vi "OEE_SCREEN_2_generate_accumulative_graph_values.vi"(11 "SCREEN_2_graph_accumulative_all_info":T1={"hour_start"=8, "hour_end"=8, "actual_by_hour"=[], "target_by_hour"=[], "X_axis_labels"=[], "SCREEN_2_graph_accumulative_references"={"graph_accumulative"=refnum, "labels_picture_accumulative"=refnum, "front_panel_reference"=refnum}}) -> (1 "Y_scale_max":dbl=160.0, 2 "Y_annotation_offset":dbl=7.9750000000000005, 3 "graph_values":cluster{dbl[], dbl[]}[](array[cluster])=[{[8.5, 9.5, 10.5, 11.5, 12.5, 13.5, 14.5, 15.5, 16.5, 17.5, 18.5, 19.5], [1.0, 5.0, 7.0, 0.0, 0.0, 0.0, 0.0, 0.0, 0.0, 0.0, 0.0, 0.0]}, {[8.5, 9.5, 10.5, 11.5, 12.5, 13.5, 14.5, 15.5, 16.5, 17.5, 18.5, 19.5], [10.0, 20.0, 30.0, 40.0, 50.0, 60.0, 70.0, 80.0, 90.0, 110.0, 120.0, 130.0]}])   [LabVIEW 2019]
uses:
  FGV/FGV_SCREEN_2_graph_accumulative/FGV_SCREEN_2_graph_accumulative_all_info.ctl
  FGV/FGV_SCREEN_2_graph_accumulative/FGV_SCREEN_2_graph_accumulative_references.ctl
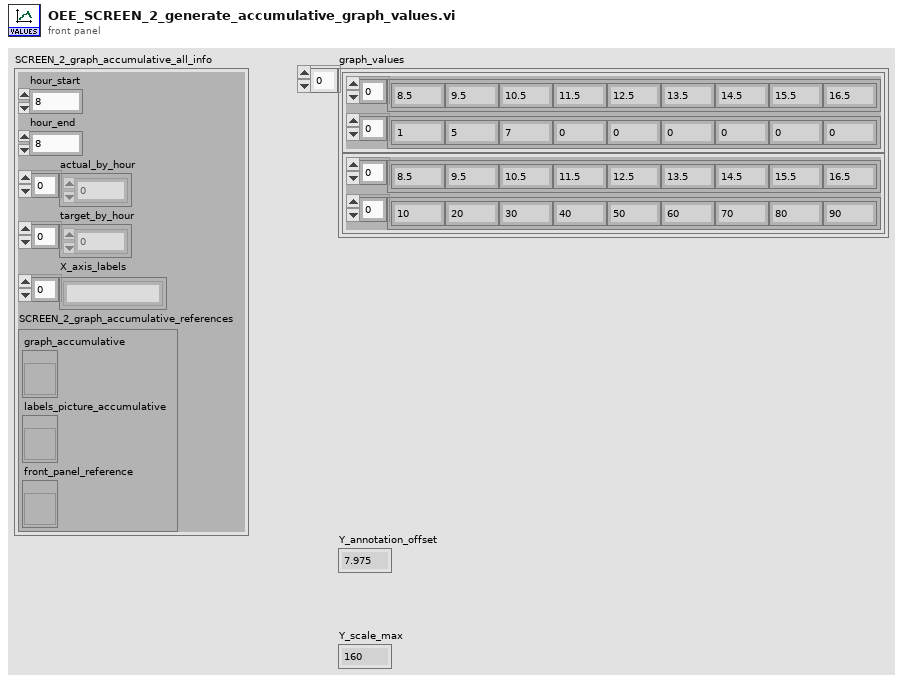
[diagram p1: front panel]
types:
  T1 = typedef "FGV_SCREEN_2_graph_accumulative_all_info.ctl" = cluster{"hour_start":i8, "hour_end":i8, "actual_by_hour":u16[], "target_by_hour":u16[], "X_axis_labels":string[], "SCREEN_2_graph_accumulative_references":T2}
  T2 = typedef "FGV_SCREEN_2_graph_accumulative_references.ctl" = cluster{"graph_accumulative":refnum<vi>, "labels_picture_accumulative":refnum<vi>, "front_panel_reference":refnum<vi>}
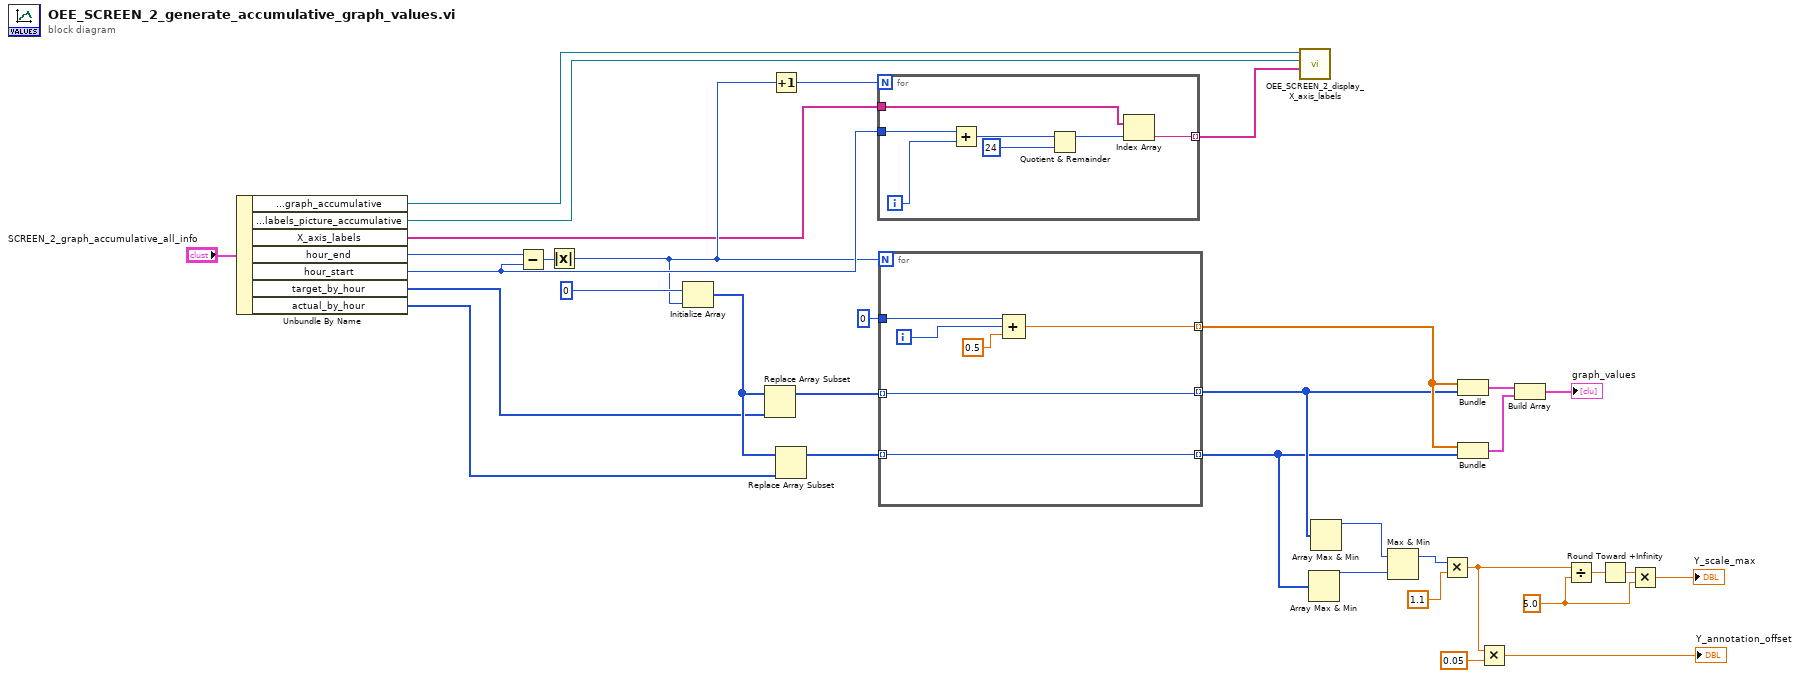
[diagram p0: block diagram]
diagram:
  w16 = 5.0 ("y")
  n1 = Unbundle By Name("SCREEN_2_graph_accumulative_all_info") -> ("SCREEN_2_graph_accumulative_references.graph_accumulative"=w7:refnum<vi>, "SCREEN_2_graph_accumulative_references.labels_picture_accumulative"=w6:refnum<vi>, "X_axis_labels"=w2:string[], "hour_end"=w10:i8, "hour_start"=w5:i8, "target_by_hour"=w9:u16[], "actual_by_hour"=w8:u16[])
  n2 = Subtract(x=w10, y=w5) -> (x-y=w12:i8)
  n3 = Absolute Value(x=w12) -> (abs(x)=w4:i8)
  n4 = Initialize Array(u16 0, w4) -> (w28:u16[])
  n5 = Replace Array Subset(array=w28, new element=w9) -> (w29:u16[])  [unwired: 1 in]
  n6 = Increment(x=w4) -> (x+1=w3:i8)
  n7 = Replace Array Subset(array=w28, new element=w8) -> (w27:u16[])  [unwired: 1 in]
  n8 = for {
    N: w3 -> [_]
    tunnel: w5 -> [w38]
    tunnel: w2 -> [w36]
    tunnel: [w35] -> w1 mode=indexing
    i -> [w37]
    n9 = Add(x=w38, y=w37) -> (x+y=w41:i32)
    n10 = Quotient & Remainder(x=w41, y=24) -> (x-y*floor(x/y)=w39:i32)  [unwired: 1 out]
    n11 = Index Array(array=w36, index=w39) -> (element=w35:string)
  }
  n12 = for {
    N: w4 -> [_]
    tunnel: u8 0 ("hour_start") -> [w47]
    tunnel: [w45] -> w31 mode=indexing
    tunnel: w29 -> [w44] mode=indexing
    tunnel: [w44] -> w20 mode=indexing
    tunnel: w27 -> [w43] mode=indexing
    tunnel: [w43] -> w19 mode=indexing
    i -> [w42]
    n13 = Compound Arithmetic op=unknown(w47, w42, 0.5 ("value")) -> (w45:dbl)
  }
  n14 = call "OEE_SCREEN_2_display_X_axis_labels.vi"("labels"=w1, "labels_picture_accumulative"=w6, "XYGraph in"=w7) -> ()  [unwired: 9 in]
  n15 = Array Max & Min(array=w19) -> (max value=w25:u16)  [unwired: 3 out]
  n16 = Array Max & Min(array=w20) -> (max value=w26:u16)  [unwired: 3 out]
  n17 = Max & Min(x=w26, y=w25) -> (max(x,y)=w24:u16)  [unwired: 1 out]
  n18 = Multiply(x=w24, y=1.1) -> (x*y=w15:dbl)
  n19 = Bundle(w31, w20) -> (w34:cluster{dbl[], u16[]})  [unwired: 1 in]
  n20 = Bundle(w31, w19) -> (w32:cluster{dbl[], u16[]})  [unwired: 1 in]
  n21 = Multiply(x=w15, y=0.05) -> (x*y=→"Y_annotation_offset":dbl)
  n22 = Build Array(w34, w32) -> (→"graph_values":cluster{dbl[], u16[]}[])
  n23 = Divide(x=w15, y=w16) -> (x/y=w18:dbl)
  n24 = Round Toward +Infinity(x=w18) -> (ceil(x): smallest int >= x=w17:dbl)
  n25 = Multiply(x=w17, y=w16) -> (x*y=→"Y_scale_max":dbl)
